vi "Init ChannelService.vi"(8 "error in (no error)":errorcluster, 11 "Vecto in":refnum<class "Vecto.lvclass">) -> (0 "error out":errorcluster, 3 "Vecto out":refnum<class "Vecto.lvclass">)   [LabVIEW 2020, in "Vecto.lvlib" / "Vecto.lvclass"]
uses:
  Vecto.lvclass
  Vecto.lvclass/Vecto.ctl
  ChannelService/ChannelService.lvclass
  Node Config/Node Config.lvclass
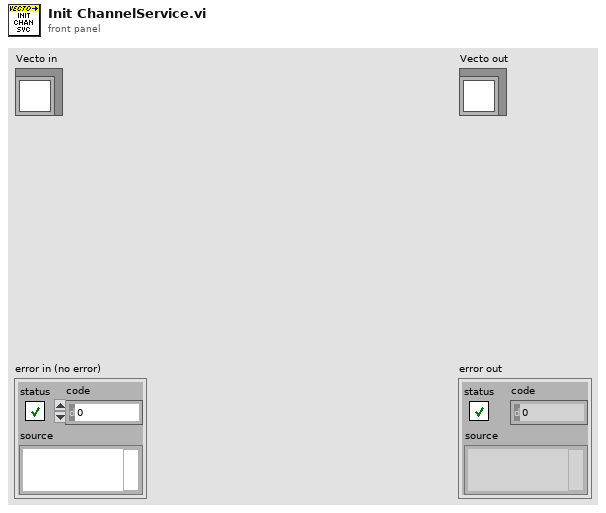
[diagram p1: front panel]
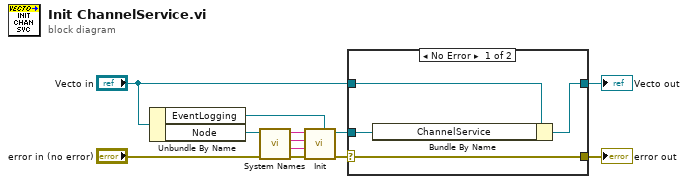
[diagram p0: block diagram]
diagram:
  n1 = Unbundle By Name("Vecto in") -> ("EventLogging"=w1:refnum<class "EventLoggingService.lvclass">, "Node"=w2:refnum<class "Node Config.lvclass">)
  n2 = call "System Names.vi"("Node Config in"=w2) -> ("Name"=w3:string, "Cluster"=w4:string, "System"=w5:string)  [unwired: 8 in]
  n3 = call "Init.vi"("EventLogger"=w1, "error in (no error)"="error in (no error)", "Node"=w3, "Cluster"=w4, "System"=w5) -> ("error out"=w10:errorcluster, "ChannelService out"=w9:refnum<class "ChannelService.lvclass">)  [unwired: 5 in]
  n4 = case shown="No Error" w10 {
    selector: w10 -> [w15 w16]
    tunnel: "Vecto in" -> [w12 w17]
    tunnel: w9 -> [w14 _]
    tunnel: [w13 w17] -> w8
    tunnel: [w15 w16] -> w7
    frame No Error {
      n5 = Bundle By Name(cluster=w12, "ChannelService"=w14) -> (w13:refnum<class "Vecto.lvclass">)
    }
    frame Error {
    }
  }
  "error out" <- w7
  "Vecto out" <- w8
